vi "NI VeriStand - Disable Dynamic Button.vi"(8 "error in (no error)":errorcluster, 11 "Button ID":string) -> (0 "error out":errorcluster)   [LabVIEW 2020, in "Custom Device API.lvlib"]
doc: "Disables a custom toolbar button for an item's <B>System Explorer</B> window configuration page. Disabled buttons do not appear in the toolbar. You can use this VI to hide a button."
uses:
  <vilib>/NI VeriStand/Custom Device API/Custom Device API.lvlib
  <vilib>/NI VeriStand/Custom Device API/Button State.ctl
  69332a04-359f-4afe-bbbc-494ca6fdc421.vi
  <vilib>/NI VeriStand/Custom Device API/Custom Device Offline Path.vi
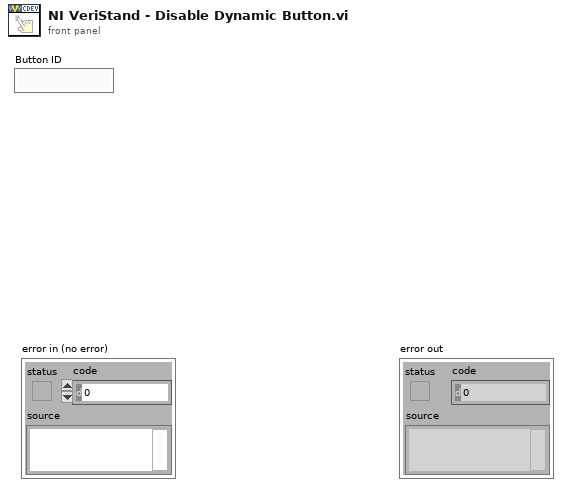
[diagram p1: front panel]
types:
  T1 = typedef "Custom Device API.lvlib/Button State.ctl" = enum16{"Enable", "Disable"}
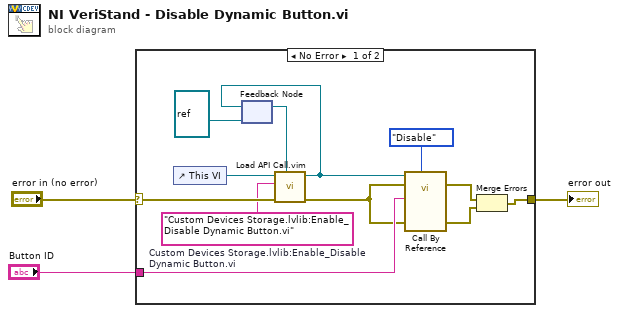
[diagram p0: block diagram]
diagram:
  n1 = case shown="No Error" "error in (no error)" {
    selector: "error in (no error)" -> [w9 w16]
    tunnel: [w14 w16] -> w3
    tunnel: "Button ID" -> [w12 _]
    frame No Error {
      w5 = "Custom Devices Storage.lvlib:Enable_Disable Dynamic Button.vi"  # Custom Devices Storage.lvlib:Enable_Disable Dynamic Button.vi
      n2 = control-ref of="This VI"() -> (w10:refnum<vi>)
      n3 = feedback #1(refnum<vi> refnum ("type specifier VI Refnum (for type only)")) -> (w11:refnum<vi>)
      n4 = call "Load API Call.vim"("VI reference in"=w11, "error in (no error)"=w9, "VI qualified name"=w5, "Caller VI ref"=w10) -> ("error out"=w8:errorcluster, "VI reference"=w7:refnum<vi>)  [unwired: 6 in]
      n5 = feedback-in #1(w7) -> ()
      n6 = call-by-ref "?"(reference=w7, error in=w8, "State"=Button_State."Disable", 8:"error in (no error)"=w8, "Button ID"=w12) -> (error out=w4:errorcluster, 0:"error out"=w15:errorcluster)  [unwired: 8 in, 1 out]
      n7 = Merge Errors(w4, w15) -> (w14:errorcluster)
    }
    frame Error {
    }
  }
  "error out" <- w3
